vi "1.3.1-Serial Read.vi"(1 "Read FIFO":refnum<k21>="Read FIFO", 5 "Receive":refnum<k21>="Port8/DIOCTL", 7 "baud rate (9600)":u32=9600, 9 "data bits (8)":i32=8 min=5 max=8 step=1, 11 "parity (0:none)":enum16{"None", "Odd", "Even", "Mark", "Space"}(ring), 12 "stop bits (10: 1 bit)":u16(ring)=10 items=["1.0"=10, "1.5"=15, "2.0"=20], 13 "Invert Polarity?":bool) -> ()   [LabVIEW 2010]
uses:
  Instance           1 27Saved   LV FPGA Serial Read .vi
  Instance           2 27Saved   LV FPGA Serial Read .vi
  <vilib>/eio/EIONode/EIONode.xnode
  Instance           3 27Saved   LV FPGA Serial Read .vi
  Instance           6 27Saved   LV FPGA Serial Read .vi
  <vilib>/rvi/DataTransferAndStorage/Container/XNode/niFpgaContainer.xnode
  <vilib>/rvi/DataTransferAndStorage/Container/Common/niFpgaContainerMethod.ctl
  <vilib>/rvi/FIFO/Fifo_Types/niFpgaFifoControlLogicControl.ctl
  <vilib>/rvi/DataTransferAndStorage/Container/Common/niFpgaContainerMetaDataKey.ctl
  <vilib>/rvi/DataTransferAndStorage/Container/Common/niFpgaContainerExecOnDevCompGetState.vi
  <vilib>/rvi/FIFO/Fifo_Resource/nirvififoEmulationSetSize.vi
  <vilib>/rvi/DataTransferAndStorage/Container/Common/niFpgaContainerGetUniqueNameForEmu.vi
  <vilib>/rvi/eio/common/nirviEmuReportErrorAndStop.vi
  <vilib>/rvi/DataTransferAndStorage/Container/Common/niFpgaTransferTypeControl.ctl
  <vilib>/rvi/interface/RandomDataEmulation/nirviRandomDataFPGAFIFO.vi
  <vilib>/rvi/interface/RandomDataEmulation/niFpgaRandomDataHandleErrors.vi
  <vilib>/rvi/DataTransferAndStorage/FIFO/niFpgaPeerToPeerStreamState.ctl
  1.0-Hindbrain Global.vi
panel:
  out "Read: Transmission Error":bool
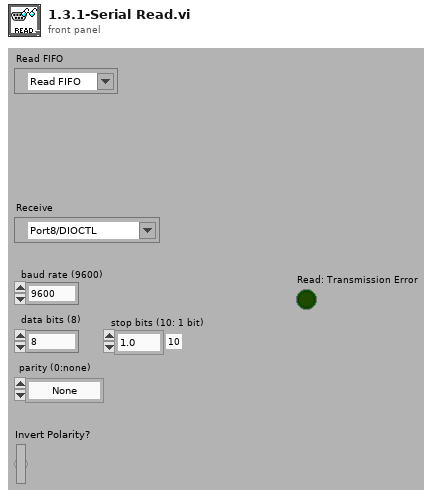
[diagram p1: front panel]
types:
  T1 = typedef "niFpgaFifoControlLogicControl.ctl" = enum16{"Slice Fabric", "Target Optimal", "Built-in"}
  T2 = typedef "niFpgaContainerMethod.ctl" = enum16{"<none>", "write", "read", "clear", "getNumberOfElementsToWrite", "getNumberOfElementsToRead", "enable", "disable", "flushAndDisable", "getStreamState", "readA", "readB", "dramWrite", "dramWriteWithByteEnables", "dramRequestData", "dramRetrieveData"}
  T3 = typedef "niFpgaTransferTypeControl.ctl" = enum16{"Target-Scoped", "Host to Target - DMA", "Target to Host - DMA", "Peer to Peer Reader", "Peer to Peer Writer", "Bidirectional"}
  T4 = typedef "niFpgaPeerToPeerStreamState.ctl" = enum16{"Unlinked", "Disabled", "Enabled", "Flushing"}
  T5 = typedef "niFpgaContainerMetaDataKey.ctl" = enum16{"FPGA FIFO", "FPGA Memory", "FPGA Register"}
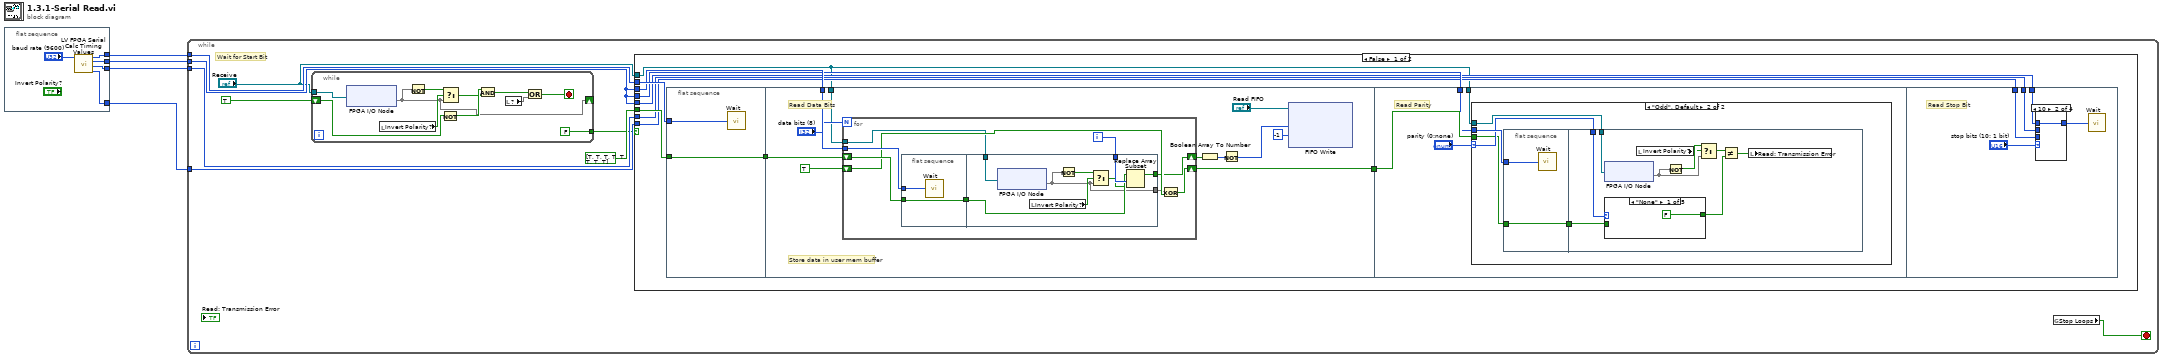
[diagram p0: block diagram]
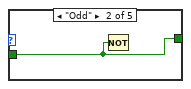
[diagram p3: hidden frame]
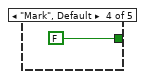
[diagram p5: hidden frame]
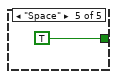
[diagram p6: hidden frame]
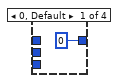
[diagram p7: hidden frame]
diagram:
  n1 = flat-sequence {
    tunnel: [w5] -> w3
    tunnel: [w8] -> w4
    tunnel: [w7] -> w2
    tunnel: [w6] -> w1
    frame #0 {
      n2 = call "LV FPGA Serial Calc Timing Values.vi"("baud rate (1000000)"="baud rate (9600)") -> ("Two Bit"=w6:u32, "One and Half Bit"=w7:u32, "One Bit"=w5:u32, "Half Bit"=w8:u32)  [unwired: 1 in, 2 out]
    }
  }
  n3 = while {
    tunnel: w1 -> [w17]
    tunnel: w2 -> [w16]
    tunnel: w3 -> [w15]
    tunnel: w4 -> [w14]
    stop <- w10 stop-if-true
    # "Wait for Start Bit"
    n4 = while {
      tunnel: [FALSE] -> w13
      shift-right: [w19] -> _
      shift-left: TRUE -> [w28]
      tunnel: "Receive" -> [w23]
      stop <- w24 stop-if-true
      n5 = xnode "FPGA I/O Node"("FPGA I/O In"=w23) -> ("I/O Item"=w19)  [unwired: 1 out]
      n6 = local read "Invert Polarity?"() -> (w21:bool)
      n7 = Not(x=w19) -> (.not. x?=w22:bool)
      n8 = Not(x=w28) -> (.not. x?=w27:bool)
      n9 = Select(t=w22, s=w21, f=w19) -> (s? t:f=w20:bool)
      n10 = And(x=w27, y=w20) -> (x .and. y?=w25:bool)
      n11 = local read item#-1() -> (w26)
      n12 = Or(x=w25, y=w26) -> (x .or. y?=w24:bool)
    }
    n13 = case shown="False" w13 {
      tunnel: bool[] [TRUE, TRUE, TRUE, TRUE, TRUE, TRUE, TRUE, TRUE] -> [w38 _]
      tunnel: w14 -> [w37 _]
      tunnel: w15 -> [w36 _]
      tunnel: w15 -> [w35 _]
      tunnel: w15 -> [w34 _]
      tunnel: w16 -> [w33 _]
      tunnel: w17 -> [w32 _]
      tunnel: "Receive" -> [w30 _]
      frame False {
        n14 = flat-sequence {
          tunnel: [w41] -> w39
          tunnel: w38 -> [w41]
          tunnel: w37 -> [w40]
          tunnel: w39 -> [w52]
          tunnel: w36 -> [w51]
          tunnel: [w47] -> w31
          tunnel: w30 -> [w45]
          tunnel: w35 -> [w390]
          tunnel: w31 -> [w392]
          tunnel: w30 -> [w389]
          tunnel: w34 -> [w417]
          tunnel: w33 -> [w416]
          tunnel: w32 -> [w415]
          frame #0 {
            n15 = call "Wait"("Count(Ticks)"=w40) -> ()  [unwired: 1 out]
          }
          frame #1 {
            # "Store data in user mem buffer"
            # "Read Data Bits"
            n16 = for {
              N: "data bits (8)" -> [_]
              shift-right: [w372] -> w50
              shift-left: w52 -> [w378]
              tunnel: w51 -> [w376]
              shift-right: [w375] -> w47
              shift-left: TRUE -> [w374]
              tunnel: w45 -> [w370]
              i -> [w371]
              n17 = flat-sequence {
                tunnel: w378 -> [w380]
                tunnel: [w380] -> w377
                tunnel: w376 -> [w379]
                tunnel: w371 -> [w388]
                tunnel: w377 -> [w387]
                tunnel: [w386] -> w372
                tunnel: [w381] -> w373
                tunnel: w370 -> [w385]
                frame #0 {
                  n18 = call "Wait"("Count(Ticks)"=w379) -> ()  [unwired: 1 out]
                }
                frame #1 {
                  n19 = xnode "FPGA I/O Node"("FPGA I/O In"=w385) -> ("I/O Item"=w381)  [unwired: 1 out]
                  n20 = local read "Invert Polarity?"() -> (w384:bool)
                  n21 = Not(x=w381) -> (.not. x?=w383:bool)
                  n22 = Select(t=w383, s=w384, f=w381) -> (s? t:f=w382:bool)
                  n23 = Replace Array Subset(array=w387, new element=w382, index=w388) -> (w386:bool[])
                }
              }
              n24 = Exclusive Or(1:w374, 2:w373) -> (0:w375:bool)
            }
            n25 = Boolean Array To Number(Boolean array=w50) -> (number=w49:u8)
            n26 = Not(x=w49) -> (.not. x?=w44:u8)
            n27 = xnode ("FIFO Write")("Element"=w44, "Timeout"=-1, "FIFO In"="Read FIFO") -> ()  [unwired: 2 out]
          }
          frame #2 {
            # "Read Parity"
            n28 = case shown="\"Odd\", Default" "parity (0:none)" {
              selector: "parity (0:none)" -> [_ w396]
              tunnel: w392 -> [_ w394]
              tunnel: w390 -> [_ w397]
              tunnel: w389 -> [_ w393]
              frame "None" {
              }
              frame "Odd", Default {
                n29 = flat-sequence {
                  tunnel: w397 -> [w399]
                  tunnel: [w398] -> w395
                  tunnel: w394 -> [w398]
                  tunnel: w396 -> [w408]
                  tunnel: w395 -> [w406]
                  tunnel: w393 -> [w404]
                  frame #0 {
                    n30 = call "Wait"("Count(Ticks)"=w399) -> ()  [unwired: 1 out]
                  }
                  frame #1 {
                    n31 = xnode "FPGA I/O Node"("FPGA I/O In"=w404) -> ("I/O Item"=w401)  [unwired: 1 out]
                    n32 = case shown="\"None\"" w408 {
                      tunnel: w406 -> [_ w410 w411 _ _]
                      tunnel: [FALSE ("y") w410 w411 FALSE ("y") TRUE ("y")] -> w407
                      frame "None" {
                      }
                      frame "Odd" {
                        n33 = Not(x=w410) -> ()  [unwired: 1 out]
                      }
                      frame "Even" {
                      }
                      frame "Mark", Default {
                      }
                      frame "Space" {
                      }
                    }
                    n34 = local read "Invert Polarity?"() -> (w402:bool)
                    n35 = Not(x=w401) -> (.not. x?=w403:bool)
                    n36 = Select(t=w403, s=w402, f=w401) -> (s? t:f=w400:bool)
                    n37 = Not Equal?(x=w400, y=w407) -> (x != y?=w405:bool)
                    n38 = local write "Read: Transmission Error"(w405) -> ()
                  }
                }
              }
            }
          }
          frame #3 {
            # "Read Stop Bit"
            n39 = case shown="10" "stop bits (10: 1 bit)" {
              tunnel: w417 -> [_ w420 _ _]
              tunnel: w416 -> [_ _ w421 _]
              tunnel: w415 -> [_ _ _ w422]
              tunnel: [u32 0 ("One Bit") w420 w421 w422] -> w414
              frame 0, Default {
              }
              frame 10 {
              }
              frame 15 {
              }
              frame 20 {
              }
            }
            n40 = call "Wait"("Count(Ticks)"=w414) -> ()  [unwired: 1 out]
          }
        }
      }
      frame True {
      }
    }
    n41 = global read "1.0-Hindbrain Global.vi" "Stop Loops"() -> (w10:bool)
  }
